vi "Word Report Mult..vi"(4 "עבר/נכשל":string="עבר/נכשל", 5 "מפעיל":string="ANS", 6 "שם הצב\"ד":string="שם הצב\"ד", 7 "מספר סידורי":string, 8 "error in (no error)":errorcluster, 9 "מק\"ט המכלל":string, 10 "Array of Items":cluster{"Details":string[][]}[](array[cluster]), 11 "Elements":string[](array[string])) -> (0 "error out":errorcluster)   [LabVIEW 2014]
uses:
  <vilib>/addons/_office/_exclsub.llb/font.ctl
  <vilib>/addons/_office/word.llb/Word Easy Table (str).vi
  <vilib>/addons/_office/word.llb/Word Edit Cell ([str]).vi
  <vilib>/addons/_office/NI_ReportGenerationToolkit.lvlib
  <vilib>/Utility/NIReport.llb/Word/NI_Word.lvclass
panel:
  in  "start (0, 0)":cluster{"row":i32, "column":i32}={"row"=1, "column"=4}
  in  "value 3":string[][](array[string])
  in  "new element/subarray 3":string[](array[string])
  in  "new element/subarray 2":string[](array[string])
  in  "value 2":string[][](array[string])
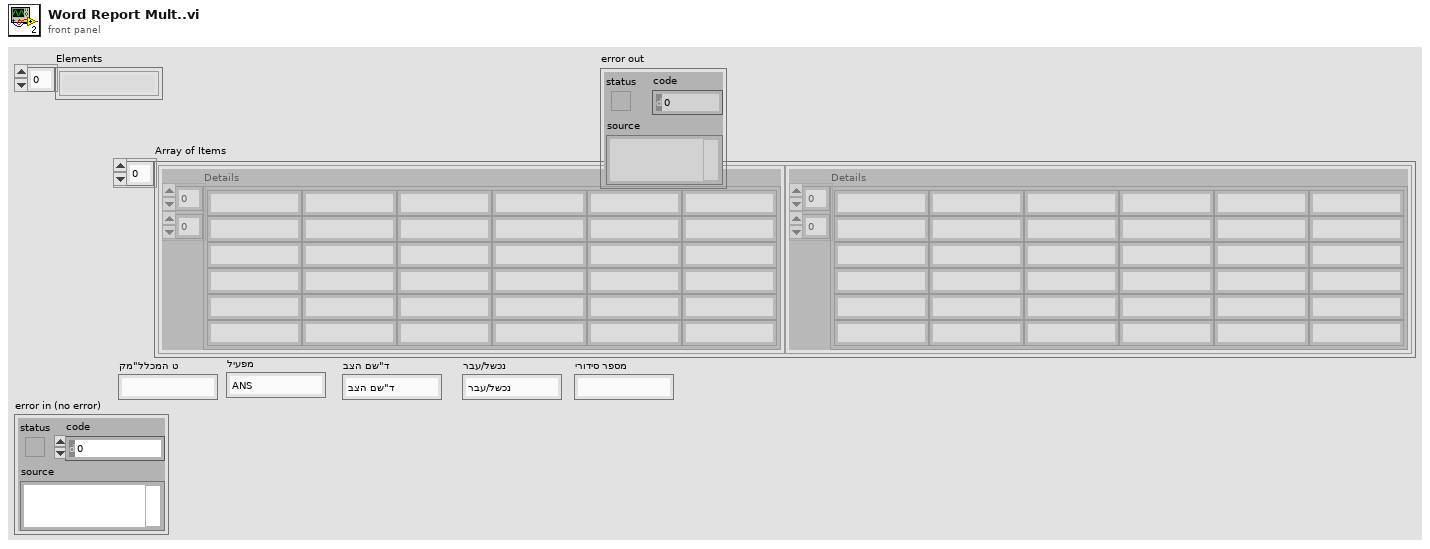
[diagram p1: front panel]
types:
  T1 = typedef "NI_ReportGenerationToolkit.lvlib/font.ctl" = cluster{"font name":string, "font size":dbl, "bold":u16, "italic":u16, "underline":u16, "strike through":u16, "font color":u32}
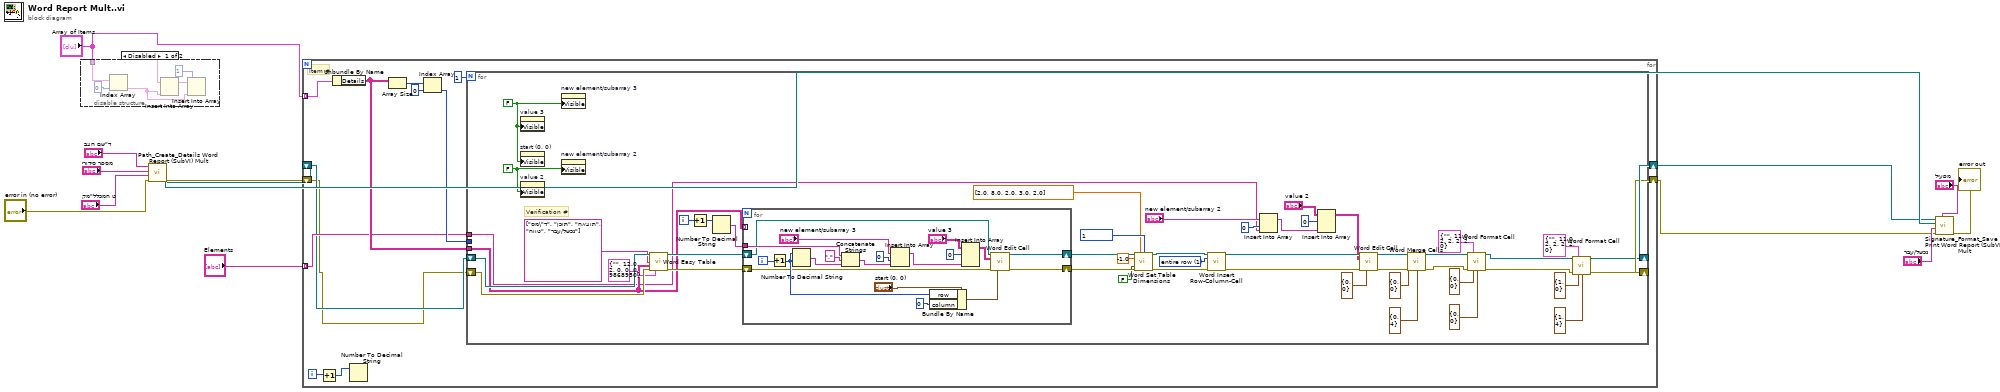
[diagram p0: block diagram]
diagram:
  n1 = disable-structure shown="Disabled" {
    disable-tunnel: "Array of Items" -> [w15 _]
    frame Disabled {
      n2 = Index Array(array=w15, index=0) -> (element=w16:cluster{"Details":string[][]})
      n3 = Insert Into Array(array=w15, new element=w16) -> (w18:cluster{"Details":string[][]}[])  [unwired: 1 in]
      n4 = Insert Into Array(array=w18, index=1, new element=w16) -> ()  [unwired: 1 out]
    }
    frame Enabled {
    }
  }
  n5 = call "Path_Create_Details Word Report (SubVI) Mult.vi"("error in (no error)"="error in (no error)", "שם ומק\"ט המכלל"="מק\"ט המכלל", "מספר סידורי"="מספר סידורי", "שם הצב\"ד"="שם הצב\"ד") -> ("error out"=w10:errorcluster, "Path"=w13:path, "NI_report out"=w9:refnum<class "NI_report.lvclass">)  [unwired: 5 in]
  n6 = for {
    shift-right: [w31] -> w7
    shift-left: w10 -> [w20]
    shift-right: [w32] -> w8
    shift-left: w9 -> [w21]
    tunnel: "Array of Items" -> [w28] mode=indexing
    tunnel: "Elements" -> [w22] mode=indexing
    i -> [w29]
    # "Item #"
    n7 = Increment(x=w29) -> (x+1=w30:i32)
    n8 = Unbundle By Name(w28) -> ("Details"=w24:string[][])
    n9 = Number To Decimal String(number=w30) -> ()  [unwired: 1 in, 1 out]
    n10 = Array Size(array=w24) -> (size(s)=w27:i32[])
    n11 = Index Array(array=w27, index=0) -> (element=w25:i32)
    n12 = for {
      N: 1 -> [_]
      shift-right: [w62] -> w31
      shift-left: w20 -> [w79]
      shift-right: [w63] -> w32
      shift-left: w21 -> [w78]
      tunnel: w22 -> [w43]
      tunnel: w25 -> [_]
      tunnel: w24 -> [w44]
      i -> [w54]
      w55 = FALSE
      w64 = FALSE
      w77 = u16 1 items=["shift cells right", "entire row", "entire column"] ("mode (entire column)")
      # "Verification #"
      n13 = property on="value 3" class="Arr (strict)"("Visible"=w55) -> ()  [unwired: 2 in, 2 out]
      n14 = property on="start (0, 0)" class="Clust (strict)"("Visible"=w55) -> ()  [unwired: 2 in, 2 out]
      n15 = property on="value 2" class="Arr (strict)"("Visible"=w64) -> ()  [unwired: 2 in, 2 out]
      n16 = property on="new element/subarray 3" class="Arr (strict)"("Visible"=w55) -> ()  [unwired: 2 in, 2 out]
      n17 = property on="new element/subarray 2" class="Arr (strict)"("Visible"=w64) -> ()  [unwired: 2 in, 2 out]
      n18 = call-poly <vilib>:"Word Easy Table.vi"("report in"=w78, "column headers"=string[] ["מס\"ד", "תוכן", "תוצאה", "טווח", "עבר/נכשל"], "data"=w44, "error in (no error)"=w79, "font"=T1 {"font name"="", "font size"=12.0, "bold"=2, "italic"=0, "underline"=0, "strike through"=0, "font color"=9868950}) -> ("report out"=w57:refnum<class "NI_report.lvclass">, "error out"=w56:errorcluster)  [unwired: 8 in, 1 out]
      n19 = Increment(x=w54) -> (x+1=w53:i32)
      n20 = Number To Decimal String(number=w53) -> (decimal integer string=w51:string)  [unwired: 1 in]
      n21 = for {
        shift-right: [w85] -> w49
        shift-left: w57 -> [w80]
        shift-right: [w84] -> w48
        shift-left: w56 -> [w81]
        tunnel: w51 -> [w89]
        tunnel: w44 -> [_] mode=indexing
        i -> [w86]
        n22 = Increment(x=w86) -> (x+1=w87:i32)
        n23 = Number To Decimal String(number=w87) -> (decimal integer string=w90:string)  [unwired: 1 in]
        n24 = Concatenate Strings(w89, ".", w90) -> (w92:string)
        n25 = Insert Into Array(array="new element/subarray 3", index=0, new element=w92) -> (w97:string[])
        n26 = Bundle By Name(cluster="start (0, 0)", "row"=w87, "column"=0) -> (w82:cluster{"row":i32, "column":i32})
        n27 = Insert Into Array(array="value 3", index (row)=0 ("disabled index (col)"), new element=w97) -> (w83:string[][])  [unwired: 1 in]
        n28 = call-poly <vilib>:"Word Edit Cell.vi"("report in"=w80, "value"=w83, "error in (no error)"=w81, "start (0, 0)"=w82) -> ("report out"=w85:refnum<class "NI_report.lvclass">, "error out"=w84:errorcluster)  [unwired: 10 in]
      }
      n29 = call <vilib>:"Word Set Table Dimensions.vi"("report in"=w49, "table column widths"=sgl[] [2.0, 8.0, 2.0, 3.0, 2.0], "measurement system"=u16 1, "left indent (0)"=sgl -1.0, "error in (no error)"=w48, "fit to page width? (F)"=FALSE) -> ("report out"=w42:refnum<class "NI_report.lvclass">, "error out"=w41:errorcluster)  [unwired: 8 in]
      n30 = call <vilib>:"Word Insert Row-Column-Cell.vi"("report in"=w42, "mode (entire column)"=w77, "error in (no error)"=w41) -> ("report out"=w70:refnum<class "NI_report.lvclass">, "error out"=w71:errorcluster)  [unwired: 11 in]
      n31 = Insert Into Array(array="new element/subarray 2", index=0, new element=w43) -> (w67:string[])
      n32 = Insert Into Array(array="value 2", index (row)=0, new element=w67) -> (w58:string[][])  [unwired: 1 in]
      n33 = call-poly <vilib>:"Word Edit Cell.vi"("report in"=w70, "value"=w58, "error in (no error)"=w71, "start (0, 0)"=cluster{"row":i32, "column":i32} {"row"=0, "column"=0}) -> ("report out"=w75:refnum<class "NI_report.lvclass">, "error out"=w76:errorcluster)  [unwired: 10 in]
      n34 = call <vilib>:"Word Merge Cells.vi"("report in"=w75, "error in (no error)"=w76, "start (0, 0)"=cluster{"start row":i32, "start column":i32} {"start row"=0, "start column"=0}, "end"=cluster{"end row":i32, "end column":i32} {"end row"=0, "end column"=4}) -> ("report out"=w37:refnum<class "NI_report.lvclass">, "error out"=w36:errorcluster)  [unwired: 10 in]
      n35 = call <vilib>:"Word Format Cell.vi"("report in"=w37, "font"=T1 {"font name"="", "font size"=11.0, "bold"=2, "italic"=2, "underline"=2, "strike through"=2, "font color"=0}, "error in (no error)"=w36, "start (-1, -1)"=cluster{"start row":i32, "start column":i32} {"start row"=0, "start column"=0}, "end (-1, -1)"=cluster{"end row":i32, "end column":i32} {"end row"=0, "end column"=0}) -> ("report out"=w34:refnum<class "NI_report.lvclass">, "error out"=w35:errorcluster)  [unwired: 9 in]
      n36 = call <vilib>:"Word Format Cell.vi"("report in"=w34, "font"=T1 {"font name"="", "font size"=11.0, "bold"=2, "italic"=2, "underline"=2, "strike through"=2, "font color"=0}, "error in (no error)"=w35, "start (-1, -1)"=cluster{"start row":i32, "start column":i32} {"start row"=1, "start column"=0}, "end (-1, -1)"=cluster{"end row":i32, "end column":i32} {"end row"=1, "end column"=4}) -> ("report out"=w63:refnum<class "NI_report.lvclass">, "error out"=w62:errorcluster)  [unwired: 9 in]
    }
  }
  n37 = call "Signature_Format_Save n Print Word Report (SubVI) Mult.vi"("מפעיל"="מפעיל", "error in (no error)"=w7, "עבר/נכשל"="עבר/נכשל", "Path"=w13, "NI_report in"=w8) -> ("error out"=→"error out":errorcluster)  [unwired: 6 in]
